vi "to_json.vi"(8 "error in":errorcluster, 11 "channelConfig in":refnum<class "channelConfig.lvclass">) -> (0 "error out":errorcluster, 2 "json":string, 3 "channelConfig out":refnum<class "channelConfig.lvclass">)   [LabVIEW 2020, in "nominal types.lvlib" / "channelConfig.lvclass"]
uses:
  channelConfig.lvclass
  channelConfig.lvclass/channelConfig.ctl
  383bacbf-beb0-46d4-b203-dcb6afdce316.vi
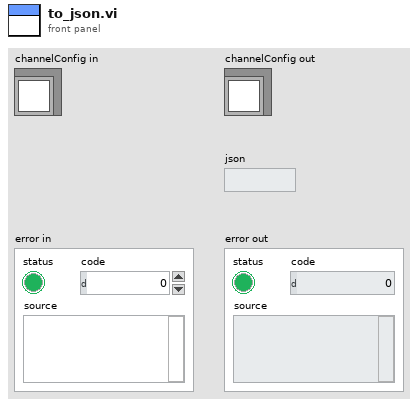
[diagram p1: front panel]
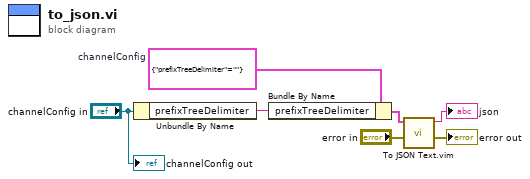
[diagram p0: block diagram]
diagram:
  w6 = cluster{"prefixTreeDelimiter":string} {"prefixTreeDelimiter"=""}  # channelConfig
  n1 = Unbundle By Name("channelConfig in") -> ("prefixTreeDelimiter"=w5:string)
  n2 = Bundle By Name(cluster=w6, "prefixTreeDelimiter"=w5) -> (w4:cluster{"prefixTreeDelimiter":string})
  n3 = call "To JSON Text.vim"("error in (no error)"="error in", "Anything"=w4) -> ("error out"=→"error out":errorcluster, "<JSON>"=→"json":string)  [unwired: 8 in]
  "channelConfig out" <- "channelConfig in"
